vi "Inst.FP.Create.vi"(8 "error in (no error)":errorcluster, 10 "FP Type":T2=enum."CF", 11 "Inst.FP in":refnum<class "Inst.FP.lvclass">) -> (0 "error out":errorcluster, 2 "Inst.FP Public Events":T1, 3 "Inst.FP out":refnum<class "Inst.FP.lvclass">)   [LabVIEW 2019, in "Inst.FP.lvclass"]
uses:
  Inst.FP.lvclass
  Typedefs/Inst.FP.Type--Enum.ctl
  C:/Program Files (x86)/National Instruments/LabVIEW 2019/user.lib/LevyLab/Instrument Framework/Instrument/Instrument.lvclass
  C:/Program Files (x86)/National Instruments/LabVIEW 2019/vi.lib/JKI/JKI SMO/SMO/SMO.lvclass
  Typedefs/PublicEvents--Cluster.ctl
  Typedefs/PublicEvents--Inst.FP.MessageFromProcess.ctl
  <userlib>/LevyLab/RemoteControl/RemoteControl/Typedefs/Message--Cluster.ctl
  <vilib>/JKI/JKI SMO/SMO/Typedefs/SMOState --Enum.ctl
  Inst.FP.lvclass/Inst.FP.ctl
  FP-TC-Shared/typedefs/LC Type--Enum.ctl
  <vilib>/JKI/JKI SMO/SMO/SMO.lvclass
  <userlib>/LevyLab/Instrument Framework/Instrument/Instrument.lvclass
  FP-TC-Shared/FP-TC-Shared.lvclass
  <userlib>/LevyLab/RemoteControl/RemoteControl/RemoteControl.lvclass
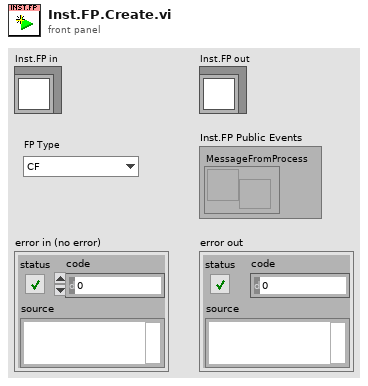
[diagram p1: front panel]
types:
  T1 = typedef "Inst.FP.lvclass/PublicEvents--Cluster.ctl" = cluster{"MessageFromProcess":refnum<user-event>}
  T2 = typedef "Inst.FP.lvclass/Inst.FP.Type--Enum.ctl" = enum32{"Wet", "CF"}
  T3 = typedef "SMO.lvclass/SMOState --Enum.ctl" = enum16{"unknown", "Created", "Started", "Stopped"}
  T4 = typedef "FP-TC-Shared.lvclass/LC Type--Enum.ctl" = enum16{"CF_FP", "CF_TC", "CF_TC_Z", "MNK_FP", "MNK_TC", "MNK_TC_Z", "unknown"}
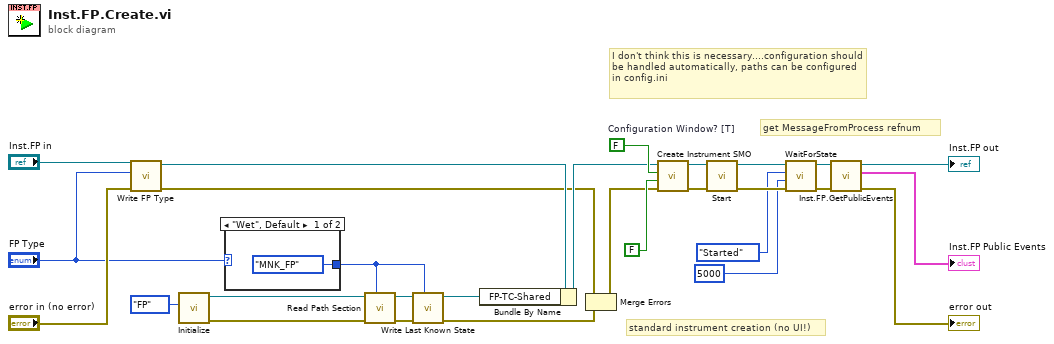
[diagram p0: block diagram]
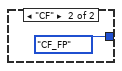
[diagram p2: hidden frame]
diagram:
  w15 = FALSE  # Configuration Window? [T]
  # "I don't think this is necessary....configuration should be handled automatically, paths can be configured in config.ini"
  # "get MessageFromProcess refnum"
  # "standard instrument creation (no UI!)"
  n1 = call "Write FP Type.vi"("error in (no error)"="error in (no error)", "FP Type"="FP Type", "Inst.FP in"="Inst.FP in") -> ("error out"=w7:errorcluster, "Inst.FP out"=w10:refnum<class "Inst.FP.lvclass">)  [unwired: 7 in]
  n2 = call "Initialize.vi"("Application"=enum16{"TC", "FP"}."FP") -> ("error out"=w4:errorcluster, "FP-TC-Shared out"=w5:refnum<class "FP-TC-Shared.lvclass">)  [unwired: 9 in]
  n3 = case shown="\"Wet\", Default" "FP Type" {
    tunnel: [LC_Type--Enum."MNK_FP" ("LC Type") LC_Type--Enum."CF_FP" ("LC Type")] -> w3
    frame "Wet", Default {
    }
    frame "CF" {
    }
  }
  n4 = call "Read Path Section.vi"("LC Type"=w3, "error in (no error)"=w4, "FP-TC-Shared in"=w5) -> ("error out"=w1:errorcluster, "FP-TC-Shared out"=w2:refnum<class "FP-TC-Shared.lvclass">)  [unwired: 6 in, 1 out]
  n5 = call "Write Last Known State.vi"("LC Type"=w3, "error in (no error)"=w1, "FP-TC-Shared in"=w2) -> ("error out"=w8:errorcluster, "FP-TC-Shared out"=w11:refnum<class "FP-TC-Shared.lvclass">)  [unwired: 7 in]
  n6 = Bundle By Name(cluster=w10, "FP-TC-Shared"=w11) -> (w9:refnum<class "Inst.FP.lvclass">)
  n7 = Merge Errors(w7, w8) -> (w6:errorcluster)
  n8 = call <userlib>:"Create Instrument SMO.vi"("error in (no error)"=w6, "Debug Mode? [F]"=FALSE, "Configuration Window? [T]"=w15, "Instrument in"=w9) -> ("error out"=w21:errorcluster, "Instrument out"=w20:refnum<class "Inst.FP.lvclass">)  [unwired: 6 in]
  n9 = call <vilib>:"Start.vi"("error in (no error)"=w21, "SMO"=w20) -> ("error out"=w26:errorcluster, "SMO out"=w23:refnum<class "Inst.FP.lvclass">)  [unwired: 8 in]
  n10 = call <vilib>:"WaitForState.vi"("error in (no error)"=w26, "timeout in ms (-1)"=5000, "State (unknown: any state)"=SMOState_--Enum."Started", "SMO in"=w23) -> ("error out"=w27:errorcluster, "SMO out"=w24:refnum<class "Inst.FP.lvclass">)  [unwired: 5 in, 1 out]
  n11 = call "Inst.FP.GetPublicEvents.vi"("error in (no error)"=w27, "Inst.FP in"=w24) -> ("error out"=→"error out":errorcluster, "Inst.FP Public Events"=→"Inst.FP Public Events":T1, "Inst.FP out"=→"Inst.FP out":refnum<class "Inst.FP.lvclass">)  [unwired: 7 in]
